vi "CtoFtemp.vi"(11 "Numeric in":dbl) -> (3 "Numeric out":dbl)   [LabVIEW 2019]
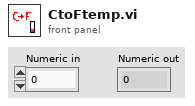
[diagram p1: front panel]
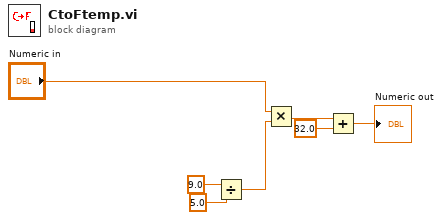
[diagram p0: block diagram]
diagram:
  n1 = Divide(x=9.0, y=5.0) -> (x/y=w3:dbl)
  n2 = Multiply(x="Numeric in", y=w3) -> (x*y=w5:dbl)
  n3 = Add(x=w5, y=32.0) -> (x+y=→"Numeric out":dbl)
